vi "add tag by line.vi"(6 "ItemNames":string[](array[string]), 8 "error in":errorcluster, 10 "TDMS datalogger configuration in":refnum<class "TDMS datalogger configuration.lvclass">, 11 "engine configuration in":refnum<class "engine configuration.lvclass">) -> (0 "error out":errorcluster, 2 "TDMS datalogger configuration out":refnum<class "TDMS datalogger configuration.lvclass">, 3 "engine configuration out":refnum<class "engine configuration.lvclass">)   [LabVIEW 2015, in "TDMS datalogger editor node.lvclass"]
uses:
  TDMS datalogger editor node.lvclass
  <vilib>/NI/Module Execution Interface/Engine Configuration/engine configuration.lvclass
  module/configuration/TDMS datalogger configuration.lvclass
  <vilib>/NI/Tag Bus/tag/Data Type.ctl
  <vilib>/NI/Configuration Framework/serializable configuration/NISE_CEF_serializable configuration.lvclass/NISE_CEF_serializable configuration.ctl
  <vilib>/NI/Tag Bus Module Framework/channel/channel classification.ctl
  <vilib>/Utility/LVClass/Get LV Class Name.vi
  <vilib>/NI/Configuration Framework/error generator/NISE_error generator.vi
  <vilib>/NI/Tag Bus/tag/tag descriptor.lvclass
  <vilib>/NI/Tag Bus Module Framework/channel/TBM channel.lvclass
  <vilib>/NI/Configuration Framework/serializable configuration/NISE_CEF_serializable configuration.lvclass
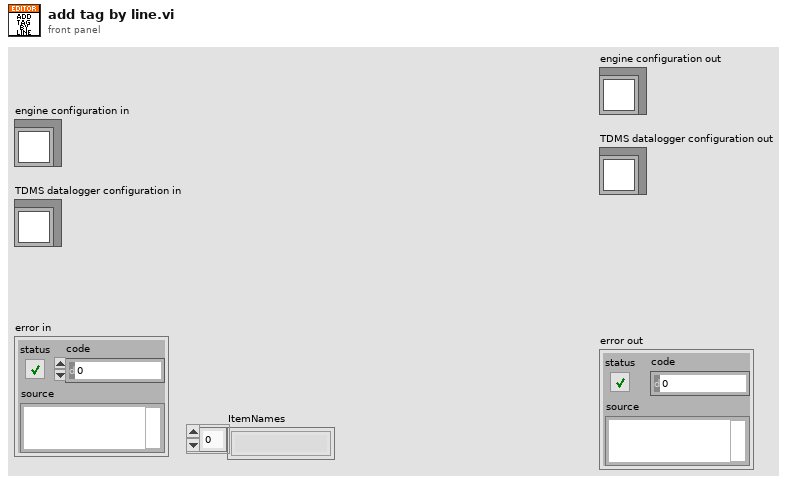
[diagram p1: front panel]
types:
  T1 = typedef "tag bus.lvlib/tag descriptor.lvclass/Data Type.ctl" = enum16{"Double", "Single", "I64", "I32", "I16", "I8", "U64", "U32", "U16", "U8", "Boolean", "String", "Array of Double", "Array of Single", "Array of I64", "Array of I32", "Array of I16", "Array of I8", "Array of U64", "Array of U32", "Array of U16", "Array of U8", "Array of Boolean", "Array of String"}
  T2 = typedef "TBM channel.lvclass/channel classification.ctl" = enum16{"input data", "output data", "processing parameter", "processing result"}
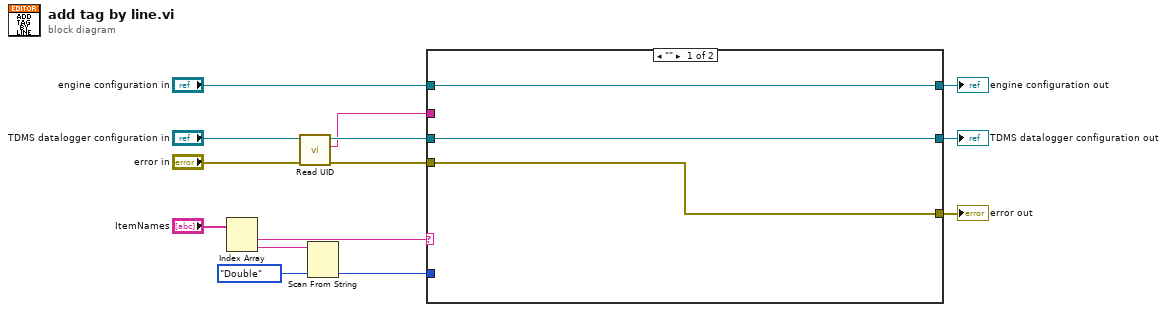
[diagram p0: block diagram]
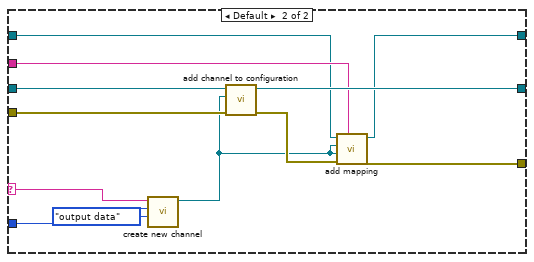
[diagram p2: hidden frame]
diagram:
  n1 = Index Array(array="ItemNames") -> (element #1=w12:string, element #2=w6:string)  [unwired: 2 in]
  n2 = call <vilib>:"Read UID.vi"("error in"="error in", "configuration in"="TDMS datalogger configuration in") -> ("error out"=w4:errorcluster, "instance id"=w1:string, "configuration out"=w2:refnum<class "TDMS datalogger configuration.lvclass">)  [unwired: 7 in]
  n3 = Scan From String(input string=w6, default 1=Data_Type."Double" ("data type")) -> (output 1=w11:T1)  [unwired: 3 in, 3 out]
  n4 = case shown="\"\"" w12 {
    selector: w12 -> [_ w29]
    tunnel: [w16 w24] -> w9
    tunnel: w2 -> [w17 w26]
    tunnel: w4 -> [w16 w25]
    tunnel: w11 -> [_ w28]
    tunnel: [w17 w23] -> w8
    tunnel: "engine configuration in" -> [w15 w19]
    tunnel: [w15 w20] -> w14
    tunnel: w1 -> [_ w21]
    frame "" {
    }
    frame Default {
      n5 = call <vilib>:"create new channel.vi"("channel classification"=channel_classification."output data", "data type"=w28, "channel name"=w29) -> ("channel"=w18:refnum<class "TBM channel.lvclass">)  [unwired: 8 in]
      n6 = call "add channel to configuration.vi"("error in"=w25, "TBM channel in"=w18, "TDMS datalogger configuration in"=w26) -> ("error out"=w22:errorcluster, "TDMS datalogger configuration out"=w23:refnum<class "TDMS datalogger configuration.lvclass">)  [unwired: 7 in]
      n7 = call <vilib>:"add mapping.vi"("owner ID"=w21, "error in"=w22, "channel"=w18, "tag descriptor"=w18, "engine configuration"=w19) -> ("error out"=w24:errorcluster, "engine configuration out"=w20:refnum<class "engine configuration.lvclass">)  [unwired: 5 in]
    }
  }
  "engine configuration out" <- w14
  "error out" <- w9
  "TDMS datalogger configuration out" <- w8
